vi "Read Snap.vi"(9 "Knob in":refnum<class "Knob.lvclass">) -> (3 "Knob out":refnum<class "Knob.lvclass">, 4 "Snap":bool)   [LabVIEW 2014, in "Knob.lvclass"]
uses:
  Knob.lvclass
  Knob.lvclass/Knob.ctl
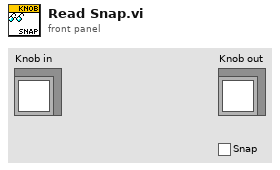
[diagram p1: front panel]
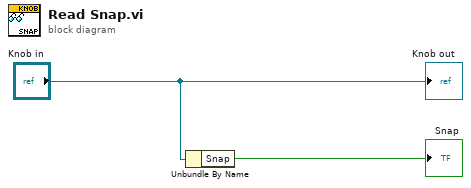
[diagram p0: block diagram]
diagram:
  n1 = Unbundle By Name("Knob in") -> ("Snap"=→"Snap":bool)
  "Knob out" <- "Knob in"
